vi "CombStage0.vi"(10 "input valid":bool, 11 "data in":bool[](array[boolean])) -> (2 "output valid":bool, 3 "data out":bool[](array[boolean]))   [LabVIEW 2011]
uses:
  <vilib>/rvi/FXPMathLib/basic elements/FxpDiscreteDelay/XNode/nifxpmath_DiscreteDelay.xnode
  <vilib>/rvi/FXPMathLib/basic elements/FxpAddSub/XNode/nifxpmath_AddSub.xnode
  <vilib>/rvi/FXPMathLib/sim/FxpSim.dll
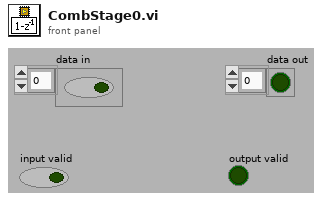
[diagram p1: front panel]
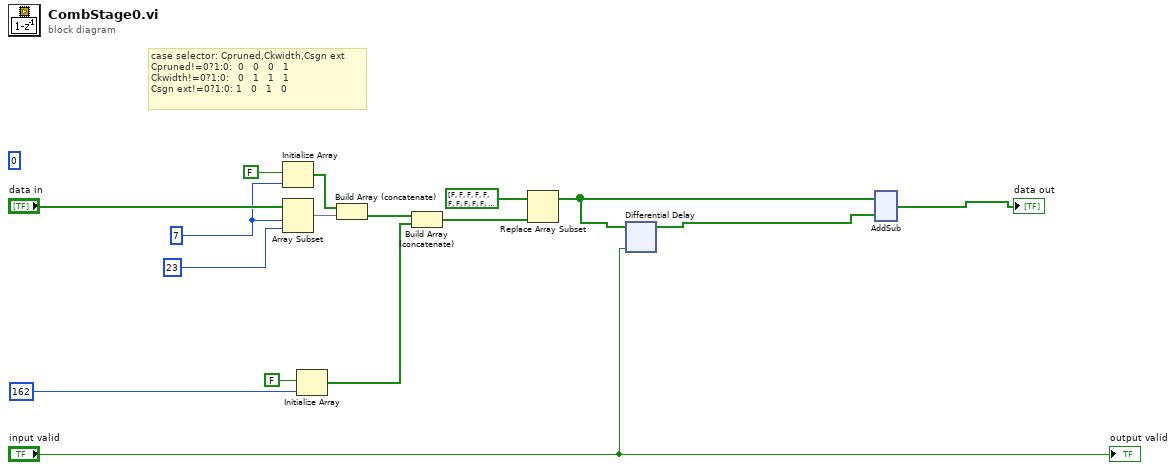
[diagram p0: block diagram]
diagram:
  w6 = 7 ("kCombPruned")
  (unwired) 0 ("kCaseSel")
  # "case selector: Cpruned,Ckwidth,Csgn ext\nCpruned!=0?1:0:  0   0   0   1\nCkwidth!=0?1:0:   0   1   1   1\nCsgn ext!=0?1:0: 1   0   1   0"
  n1 = Initialize Array(FALSE, w6) -> (w7:bool[])
  n2 = Array Subset(array="data in", index=w6, length=23 ("kCombWidth")) -> (w9:bool[])
  n3 = Initialize Array(FALSE, 162 ("kComb192-MaxWidth")) -> (w12:bool[])
  n4 = Build Array (concatenate)(w7, w9) -> (w13:bool[])
  n5 = Build Array (concatenate)(w13, w12) -> (w10:bool[])
  n6 = Replace Array Subset(array=bool[] [FALSE, FALSE, FALSE, FALSE, FALSE, FALSE, FALSE, FALSE, FALSE, FALSE, FALSE, FALSE, FALSE, FALSE, FALSE, FALSE, FALSE, FALSE, FALSE, FALSE, FALSE, FALSE, FALSE, FALSE, FALSE, FALSE, FALSE, FALSE, FALSE, FALSE, FALSE, FALSE, FALSE, FALSE, FALSE, FALSE, FALSE, FALSE, FALSE, FALSE, FALSE, FALSE, FALSE, FALSE, FALSE, FALSE, FALSE, FALSE, FALSE, FALSE, FALSE, FALSE, FALSE, FALSE, FALSE, FALSE, FALSE, FALSE, FALSE, FALSE, FALSE, FALSE, FALSE, FALSE, FALSE, FALSE, FALSE, FALSE, FALSE, FALSE, FALSE, FALSE, FALSE, FALSE, FALSE, FALSE, FALSE, FALSE, FALSE, FALSE, FALSE, FALSE, FALSE, FALSE, FALSE, FALSE, FALSE, FALSE, FALSE, FALSE, FALSE, FALSE, FALSE, FALSE, FALSE, FALSE, FALSE, FALSE, FALSE, FALSE, FALSE, FALSE, FALSE, FALSE, FALSE, FALSE, FALSE, FALSE, FALSE, FALSE, FALSE, FALSE, FALSE, FALSE, FALSE, FALSE, FALSE, FALSE, FALSE, FALSE, FALSE, FALSE, FALSE, FALSE, FALSE, FALSE, FALSE, FALSE, FALSE, FALSE, FALSE, FALSE, FALSE, FALSE, FALSE, FALSE, FALSE, FALSE, FALSE, FALSE, FALSE, FALSE, FALSE, FALSE, FALSE, FALSE, FALSE, FALSE, FALSE, FALSE, FALSE, FALSE, FALSE, FALSE, FALSE, FALSE, FALSE, FALSE, FALSE, FALSE, FALSE, FALSE, FALSE, FALSE, FALSE, FALSE, FALSE, FALSE, FALSE, FALSE, FALSE, FALSE, FALSE, FALSE, FALSE, FALSE, FALSE, FALSE, FALSE, FALSE, FALSE, FALSE, FALSE, FALSE, FALSE, FALSE, FALSE, FALSE, FALSE, FALSE, TRUE, TRUE] ("Array"), new element=w10) -> (w2:bool[])  [unwired: 1 in]
  n7 = xnode ("Differential Delay")("D"=w2, "enable"="input valid") -> ("Q"=w1:bool[])
  n8 = xnode ("AddSub")("x"=w2, "y"=w1) -> ("s"=→"data out":bool[])  [unwired: 1 out]
  "output valid" <- "input valid"
